vi "Untitled 1.vi"() -> ()   [LabVIEW 2016]
uses:
  Workspace/Workspace.ctl
  Workspace/Carrier Tray/Syringe Space/Syringe Space.lvclass
  Controller/Controller.lvclass
  Controller/Motion/Motion.lvclass
  Dispense.lvclass
  Workspace/Fixture.lvclass
panel:
  out "Workspace":T1
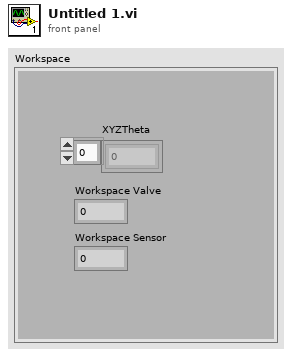
[diagram p1: front panel]
types:
  T1 = typedef "Fixture.lvclass/Workspace.ctl" = cluster{"XYZTheta":dbl[], "Workspace Valve":i32, "Workspace Sensor":i32}
  T2 = typedef "Controller.lvclass/Controllers.ctl" = cluster{"I-O.lvclass":refnum<class "I-O.lvclass">, "Motion.lvclass":refnum<class "Motion.lvclass">, "Dispenser.lvclass":refnum<class "Dispenser.lvclass">}
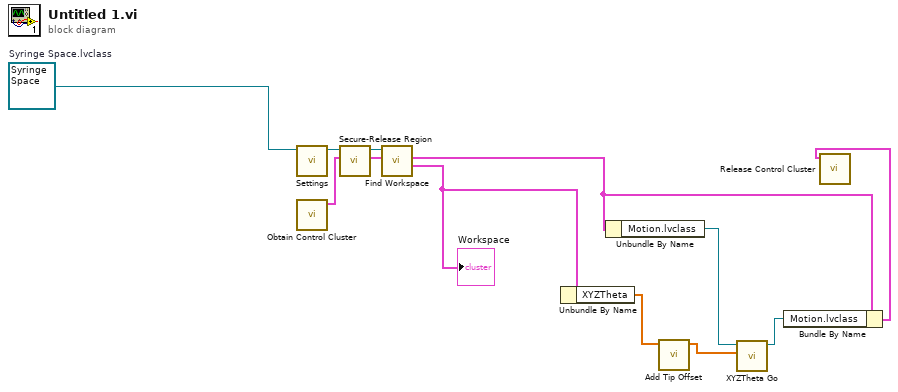
[diagram p0: block diagram]
diagram:
  w8 = refnum<class "Syringe Space.lvclass"> refnum  # Syringe Space.lvclass
  n1 = call-dynamic "Settings.vi"("Syringe Space in"=w8) -> ("Syringe Space out"=w12:refnum<class "Syringe Space.lvclass">)  [unwired: 9 in, 1 out]
  n2 = call "Obtain Control Cluster.vi"() -> ("Control Out"=w10:T2)  [unwired: 11 in]
  n3 = call-dynamic "Secure-Release Region.vi"("Control In"=w10, "Baseplate Tray in"=w12) -> ("Control Out"=w9:T2, "Baseplate Tray out"=w11:refnum<class "Syringe Space.lvclass">)  [unwired: 7 in, 1 out]
  n4 = call-dynamic "Find Workspace.vi"("Control In"=w9, "Baseplate Tray in"=w11) -> ("Workspace"=w7:T1, "Control Out"=w2:T2)  [unwired: 6 in, 2 out]
  "Workspace" <- w7
  n5 = Unbundle By Name(w7) -> ("XYZTheta"=w5:dbl[])
  n6 = Unbundle By Name(w2) -> ("Motion.lvclass"=w6:refnum<class "Motion.lvclass">)
  n7 = call "Add Tip Offset.vi"("XYZTheta"=w5) -> ("XYZTheta"=w4:dbl[])  [unwired: 10 in]
  n8 = call "XYZTheta Go.vi"("XYZTheta In"=w4, "Motion in"=w6) -> ("Motion out"=w3:refnum<class "Motion.lvclass">)  [unwired: 7 in, 2 out]
  n9 = Bundle By Name(cluster=w2, "Motion.lvclass"=w3) -> (w1:T2)
  n10 = call "Release Control Cluster.vi"("output cluster"=w1) -> ()  [unwired: 11 in]
